vi "pulse detector on usrp host.vi"() -> ()   [LabVIEW 2021]
doc: "This template is for the Simple NI-USRP Streaming design, a design that shows the basics of streaming data to and from an NI USRP-294x/295x device. Refer to the block diagram for more information about how to use this template."
uses:
  FPGA/reciver params.ctl
  Host/SubVIs/Start Trigger.ctl
  <vilib>/userDefined/Silver/nirio_resource_slv.ctl
  Host/SubVIs/Streaming Xvcr FPGA Ref.ctl
  FPGA/PDW interpoter params.ctl
  Host/SubVIs/Initiate and Fetch (Multi).vi
  Host/SubVIs/Initiate and Fetch Time (Multi).vi
  Host/SubVIs/Initiate and Trigger.vi
  Host/SubVIs/Fetch Rx Data.vi
  Host/SubVIs/Fetch Rx Data (CDB WDT).vi
  Host/SubVIs/Check Aurora Link.vi
  Host/SubVIs/Check Stream Status.vi
  <vilib>/Utility/error.llb/Error Cluster From Error Code.vi
  <vilib>/rvi/errors/niLvFpgaAdjustHostInterfaceError.vi
  <vilib>/rvi/interface/nirviMethod/nirviMethod.xnode
  <vilib>/rvi/interface/nirviReadWriteControl/nirviReadWriteControl.xnode
  <vilib>/FPGAPlugInAG/Dynamic/niLvFpga_ReadFifo_Dynamic.vi
  <vilib>/rvi/errors/niLvFpgaMergeErrorWithErrorCode.vi
  NiFpgaLv.dll
  <vilib>/rvi/interface/Simulation/niFpgaSimulationCallBeginRW.vi
panel:
  in  "Tab Control":enum32{"sumorry", "Rx graphs"}(tab)
  in  "detection bar (dB)":dbl format="%#_3p"
  out "amp(dB)/ frequncy (Hz)":cluster{dbl[], dbl[]}(graph)
  out "amp(dB)":cluster{dbl[], dbl[]}(graph)
  out "F (Hz)":cluster{dbl[], dbl[]}(graph)
  out "PW":cluster{dbl[], dbl[]}(graph)
  out "mun of polses detected":i32
  out "spots from start":i32
  out "pulse rate (PPS)":dbl format="%#_6p"
  in  "base frequnce showen":bool
  in  "sample rate":dbl=200000000.0 format="%#_6p"
  in  "frequency":dbl=800000000.0 format="%#_6p"
  in  "pre amp":dbl=30.0
  in  "PW low bar":dbl
  in  "min AMP":dbl format="%#_3p"
  in  "Pw high bar":dbl=30000.0 format="%#_3g"
  in  "lo likege removal (#of bins)":i32
  out "PW_resolotion":dbl format="%#_6p"
  out "frequncy resolotion":dbl format="%#_3p"
  in  "reciver_params":T1={"min PW (fft cycels)"=0, "max PW (fft cycels)"=1500, "max gap (fft cycels)"=0, "detection bar (liniar amp)"=93.0, "peak detect"=FALSE}
  out "acquiring":bool caption="Streaming"
  in  "Stop":bool
  # "pulse detector on usrp"
  # "this application runs the pulse detector on the IQ stream inside the USRP.\nset the parameters and run it.\nthe reciver params are the parameters needed for the pulse detector:\n max gap - the maxiemom of undetected parts in the spot that \nthe detector keep loking for continuety.\nRx max PW - if the pulse is CW then we like to get  a PDW even if the pulse isnt done.\nRx min PW - less then this size is probbly just termal noise\nRx detection bar - the detection bar.\ndisplay filters could help the user make the presenting graphs easyer to understend."
  # "user filter"
  # "USRP setup"
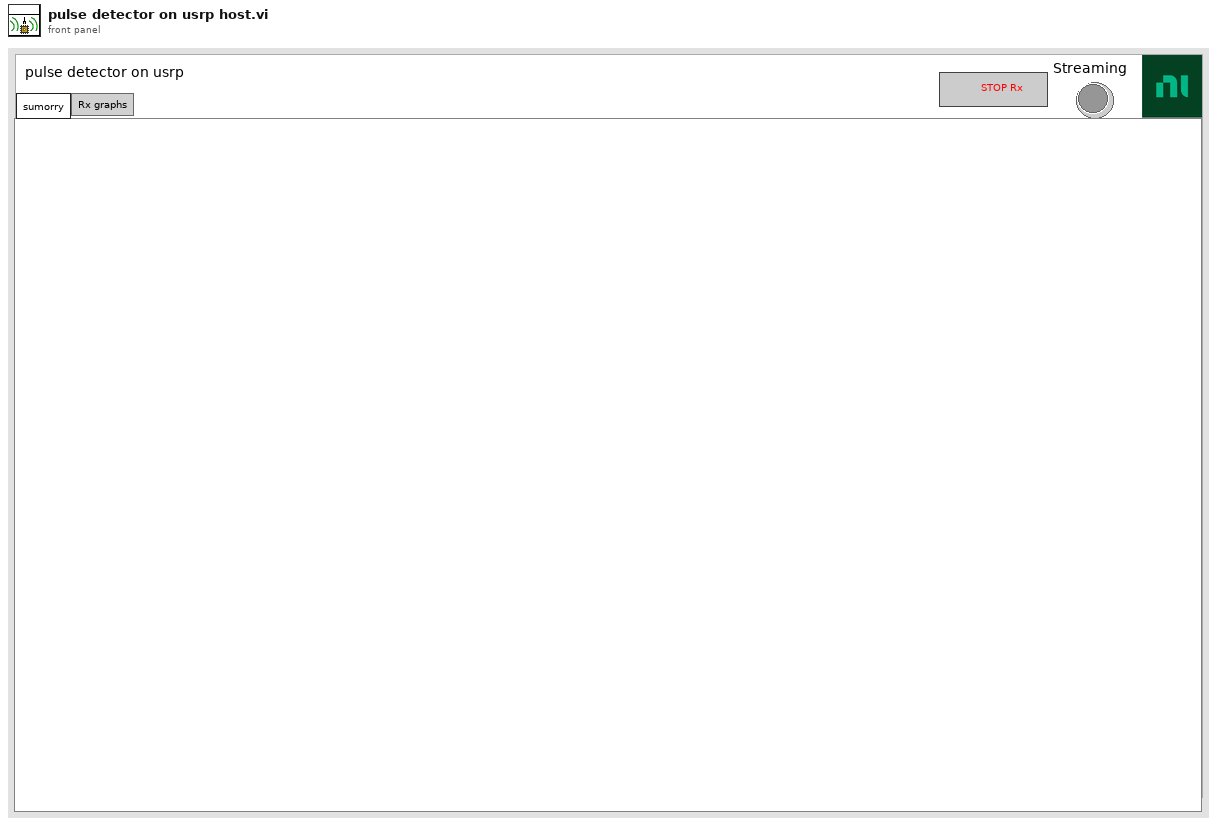
[diagram p1: front panel]
types:
  T1 = typedef "reciver params.ctl" = cluster{"min PW (fft cycels)":u16, "max PW (fft cycels)":u16, "max gap (fft cycels)":u8, "detection bar (liniar amp)":fxp<+,64,63>, "peak detect":bool}
  T2 = typedef "nirio_resource_slv.ctl" = tag
  T3 = typedef "Start Trigger.ctl" = enum8{"Software", "Digital Edge", "Rx Start Trigger", "Tx Start Trigger", "Immediate", "Future Time Event"}
  T4 = cluster{"rf enable 0":bool, "rf config 0":cluster{"antenna":string, "frequency":dbl, "lo frequency":dbl, "level":dbl}, "rf enable 1":bool, "rf config 1":cluster{"antenna":string, "frequency":dbl, "lo frequency":dbl, "level":dbl}, "transfer mode":enum16{"Finite", "Continuous"}, "sample rate":dbl, "number of samples":u32, "start trigger":T3}
  T5 = enum16{"open", "open or create", "create or replace", "create", "open (read-only)"}
  T6 = typedef "Rx Channels.ctl" = cluster{"rx config":cluster{"channel configuration":cluster{"channel enable":bool, "channel configuration":cluster{"antenna":string, "frequency":dbl, "lo frequency":dbl, "level":dbl}}[], "transfer mode":enum16{"Finite", "Continuous"}, "sample rate":dbl, "number of samples":u32, "start trigger":T3}, "reference frequency source":string, "rx.data sink":enum16{"SFP Port 0", "SFP Port 1", "Host"}, "rx.enabled channels":string[], "vertical range":dbl[], "rx.coerced configurations":cluster{"coerced frequencies":dbl[], "coerced lo frequencies":dbl[], "coerced levels":dbl[], "coerced sample rates":dbl[]}}
  T7 = typedef "niUsrpRio Config v1 Host.lvlib/niUsrpRio Session.ctl" = cluster{"FPGA Interface":refnum<k20>, "RIO Interface Number":u32, "Data Clock Rate":u32, "FPGA Data Clock Rate":u32, "Global Settings Register Bus":T8, "Radio 0 Settings Register Bus":T8, "Radio 1 Settings Register Bus":T8, "Radio Settings Bus Semaphore":T9, "DB Queues":T10[], "Characterization Data Valid?":bool, "EEPROM Header":T11, "Device Data Header":T12, "EEPROM Characterization Header":T13, "Characterization Data":T14[], "FPGA Current Version":u32, "FPGA Oldest Compatible Version":u32, "Fixed Logic Current Version":u32, "Fixed Logic Oldest Compatible Version":u32, "FPGA Radio Settings Bus Current Version":u32, "FPGA Radio Settings Bus Oldest Compatible Version":u32, "FPGA Board Config Current Version":u32, "FPGA Board Config Oldest Compatible Version":u32, "Daughterboard Clock Rate":u32, "daughterboard configuration session handles":u64[]}
  T8 = typedef "niInstr Register Bus v0 Host.lvlib/Register Bus Session.ctl" = refnum<queue>
  T9 = typedef "Semaphore RefNum" = refnum<k1>
  T10 = typedef "niUsrpRio Config v1 Host.lvlib/DB Queue Reference.ctl" = refnum<queue>
  T11 = typedef "niUsrpRio Config v1 Host.lvlib/EEPROM Header.ctl" = cluster{"Checksum":u32, "Product Code":u16, "Hardware Current Version":u16, "Hardware Oldest Compatible Version":u16, "EEPROM Map Current Version":u16, "EEPROM Map Oldest Compatible Version":u16, "User Password":string, "Pointer to Factory Header":u32, "Pointer to User Header":u32, "Recommended Interval":u16, "Number of Reserved Bytes":i32, "Number of Daughterboards":u8, "Daughterboard IDs":u16[], "Daughterboard Serial Numbers":string[]}
  T12 = typedef "niUsrpRio Config v1 Host.lvlib/EEPROM Device Data Header.ctl" = cluster{"Checksum":u32, "Number of Channels":u8, "Number of Gain Settings":u16[], "Pointer to Characterization Data":u32[], "Number of Reserved Bytes":i32, "Number of Frequencies":u16[]}
  T13 = typedef "niUsrpRio Config v1 Host.lvlib/EEPROM Characterization Header.ctl" = cluster{"Checksum":u32, "Date":timestamp, "Temperature":sgl, "Misc. Info":string, "Pointer to Device Data Header":u32, "Number of Reserved Bytes":i32}
  T14 = typedef "niUsrpRio Config v1 Host.lvlib/Characterization Data.ctl" = cluster{"Gains[dB]":dbl[], "Frequencies [Hz]":dbl[], "IQ Imbalance Table":T15[], "Measured Gains[dB]":dbl[][]}
  T15 = typedef "niUsrpRio Config v1 Host.lvlib/IQ Imbalance.ctl" = cluster{"Gain Imbalance [linear]":dbl, "Phase Imbalance [radians]":dbl, "Offset":cdb}
  T16 = typedef "PDW interpoter params.ctl" = cluster{"Fs (Hz)":u32, "fft size ":u32, "F base (Hz)":u32, "min AMP (dB)":dbl, "PW low bar (fft cycle)":dbl, "Pw high bar (fft cycle)":dbl, "lo likege removal (fft bin)":i32, "max gap (fft cycle)":dbl}
  T17 = typedef "Streaming Xvcr FPGA Ref.ctl" = refnum<k20>
  T18 = cluster{"rx.state":enum16{"Idle", "Active"}, "rx.samples processed":u32, "rx.number of fifo overflows":u32, "rx.number of iq data overflows":u64[], "rx.dsp reset done":bool}
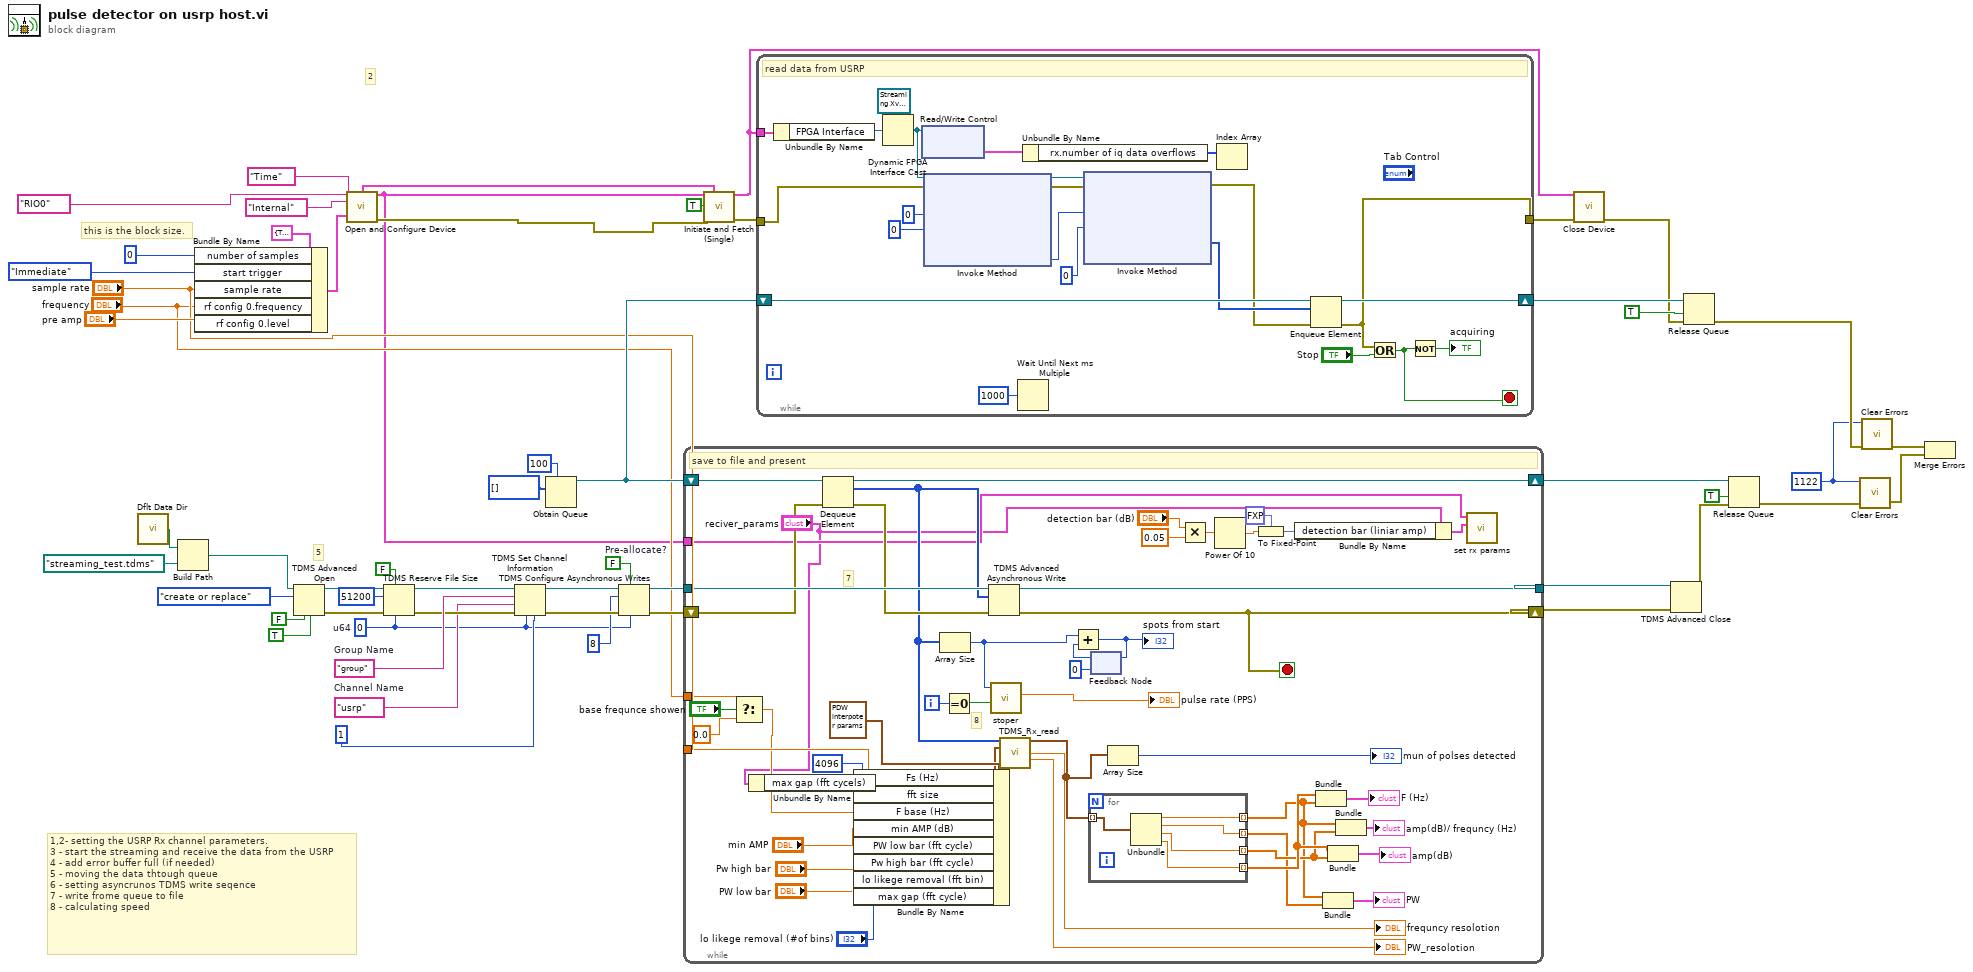
[diagram p0: block diagram]
diagram:
  w22 = 1122 ("specific error code to clear (0: all)")
  w46 = FALSE  # Pre-allocate?
  w37 = u64 0  # u64
  w55 = "group"  # Group Name
  w39 = "usrp"  # Channel Name
  # "2"
  # "this is the block size."
  # "1,2- setting the USRP Rx channel parameters.\n3 - start the streaming and receive the data from the USRP\n4 - add error buffer full (if needed)\n5 - moving the data thtough queue   \n6 - setting asyncrunos TDMS write seqence\n7 - write frome queue to file\n8 - calculating speed"
  # "5"
  n1 = call <vilib>:"Dflt Data Dir.vi"() -> ("App:Default Data Directory"=w32:path)
  n2 = Build Path(base path=w32, name or relative path=path "streaming_test.tdms") -> (appended path=w31:path)
  n3 = Bundle By Name(cluster=T4 {"rf enable 0"=TRUE, "rf config 0"={"antenna"="RX1", "frequency"=2000000000.0, "lo frequency"=-1.0, "level"=0.0}, "rf enable 1"=FALSE, "rf config 1"={"antenna"="RX2", "frequency"=2000000000.0, "lo frequency"=-1.0, "level"=0.0}, "transfer mode"=enum."Continuous", "sample rate"=10000000.0, "number of samples"=4194304, "start trigger"=enum."Immediate"} ("rx config"), "number of samples"=0, "start trigger"=Start_Trigger."Immediate", "sample rate"="sample rate", "rf config 0.frequency"="frequency", "rf config 0.level"="pre amp") -> (w15:T4)
  n4 = TDMS Advanced Open(4:TRUE ("enable asynchronous? (T)"), 6:FALSE ("disable buffering? (T)"), 10:T5."create or replace" ("operation (0:open)"), 11:w31) -> (0:w51:errorcluster, 3:w52:refnum<k34>)  [unwired: 1 in, 1 out]
  n5 = call "Open and Configure Device.vi"("USRP RIO Device"=T2 "RIO0" ("USRP RIO device"), "reference frequency source"="Internal", "which bitfile"="Time", "rx config"=w15) -> ("rx channels"=w8:T6, "niUsrpRio Session (out)"=w1:T7, "error out"=w2:errorcluster)  [unwired: 5 in, 4 out]
  n6 = TDMS Reserve File Size(6:w37, 7:FALSE ("append? (T)"), 8:w51, 10:u64 51200 ("reserve size"), 11:w52) -> (0:w49:errorcluster, 3:w50:refnum<k34>)
  n7 = TDMS Set Channel Information(4:u32 1 ("y"), 6:w37, 8:w49, 9:w39, 10:w55, 11:w50) -> (0:w48:errorcluster, 3:w47:refnum<k34>)  [unwired: 1 in]
  n8 = Obtain Queue(max queue size (-1, unlimited)=100, element data type=u64[] [] ("waveform data")) -> (queue out=w23:refnum<queue>)  [unwired: 3 in, 2 out]
  n9 = TDMS Configure Asynchronous Writes(6:w37, 7:w46, 8:w48, 10:u32 8 ("max asynchronous writes (4)"), 11:w47) -> (0:w40:errorcluster, 3:w43:refnum<k34>)  [unwired: 2 in]
  n10 = while {
    tunnel: w43 -> [w103]
    shift-right: [w99] -> w41
    shift-left: w23 -> [w104]
    tunnel: [w101] -> w42
    shift-right: [w102] -> w35
    shift-left: w40 -> [w98]
    tunnel: "sample rate" -> [w69]
    tunnel: "frequency" -> [w67]
    tunnel: w1 -> [w60]
    i -> [w100]
    stop <- w102 stop-if-true
    # "8"
    # "7"
    # "save to file and present"
    n11 = Select(t=w67, s="base frequnce showen", f=0.0) -> (s? t:f=w68:dbl)
    n12 = Unbundle By Name("reciver_params") -> ("max gap (fft cycels)"=w74:u8)
    n13 = Dequeue Element(queue=w104, error in (no error)=w98) -> (queue out=w99:refnum<queue>, element=w79:u64[], error out=w97:errorcluster)  [unwired: 1 in, 1 out]
    n14 = Bundle By Name(cluster=T16 {"Fs (Hz)"=200000000, "fft size "=4096, "F base (Hz)"=2000000000, "min AMP (dB)"=0.0, "PW low bar (fft cycle)"=0.0, "Pw high bar (fft cycle)"=7000.0, "lo likege removal (fft bin)"=-1, "max gap (fft cycle)"=0.0} ("PDW interpoter params"), "Fs (Hz)"=w69, "fft size"=u32 4096, "F base (Hz)"=w68, "min AMP (dB)"="min AMP", "PW low bar (fft cycle)"="PW low bar", "Pw high bar (fft cycle)"="Pw high bar", "lo likege removal (fft bin)"="lo likege removal (#of bins)", "max gap (fft cycle)"=w74) -> (w76:T16)
    n15 = Array Size(array=w79) -> (size(s)=w94:i32)
    n16 = Equal To 0?(x=w100) -> (x = 0?=w96:bool)
    n17 = TDMS Advanced Asynchronous Write(8:w97, 10:w79, 11:w103) -> (0:w102:errorcluster, 3:w101:refnum<k34>)
    n18 = call "stoper.vi"("start"=w96, "x mission"=w94) -> ("x rate"=→"pulse rate (PPS)":dbl)  [unwired: 7 in, 2 out]
    n19 = call "TDMS_Rx_read.vi"("Array in"=w79, "PDW interpoter params"=w76) -> ("Array"=w80:cluster{dbl, dbl, "fixed-point":dbl, dbl}[], "frequncy resolotion"=→"frequncy resolotion":dbl, "PW_resolotion"=→"PW_resolotion":dbl)  [unwired: 11 in]
    n20 = for {
      tunnel: w80 -> [w109] mode=indexing
      tunnel: [w108] -> w78 mode=indexing
      tunnel: [w107] -> w81 mode=indexing
      tunnel: [w106] -> w82 mode=indexing
      tunnel: [w105] -> w83 mode=indexing
      n21 = Unbundle(w109) -> (w108:dbl, w107:dbl, "fixed-point"=w106:dbl, w105:dbl)
    }
    n22 = feedback #1(0) -> (w92:i32)
    n23 = Add(x=w94, y=w92) -> (x+y=w93:i32)
    "spots from start" <- w93
    n24 = feedback-in #1(w93) -> ()
    n25 = Array Size(array=w80) -> (size(s)=→"mun of polses detected":i32)
    n26 = Multiply(x="detection bar (dB)", y=0.05) -> (x*y=w61:dbl)
    n27 = Power Of 10(x=w61) -> (10^x=w62:dbl)
    n28 = To Fixed-Point(fixed-point type=fxp<+,64,63> 0.0 ("detection bar (liniar amp)"), number=w62) -> (fixed-point=w63:fxp<+,64,63>)
    n29 = Bundle By Name(cluster="reciver_params", "detection bar (liniar amp)"=w63) -> (w64:T1)
    n30 = Bundle(w83, w78) -> (→"F (Hz)":cluster{dbl[], dbl[]})  [unwired: 1 in]
    n31 = Bundle(w78, w81) -> (→"PW":cluster{dbl[], dbl[]})  [unwired: 1 in]
    n32 = Bundle(w83, w82) -> (→"amp(dB)":cluster{dbl[], dbl[]})  [unwired: 1 in]
    n33 = Bundle(w78, w82) -> (→"amp(dB)/ frequncy (Hz)":cluster{dbl[], dbl[]})  [unwired: 1 in]
    n34 = call "set rx params.vi"("reciver_params"=w64, "niUsrpRio Session (out)"=w60) -> ()  [unwired: 8 in, 2 out]
  }
  n35 = call "Initiate and Fetch (Single).vi"("niUsrpRio Session"=w1, "rx channels"=w8, "first iteration"=TRUE, "error in"=w2) -> ("niUsrpRio Session (out)"=w7:T7, "error out"=w6:errorcluster)  [unwired: 9 in, 1 out]
  n36 = while {
    shift-right: [w131] -> w29
    shift-left: w23 -> [w130]
    tunnel: [w126] -> w13
    tunnel: w7 -> [w121]
    tunnel: w6 -> [w113]
    stop <- w127 stop-if-true
    # "read data from USRP"
    n37 = Unbundle By Name(w121) -> ("FPGA Interface"=w125:refnum<k20>)
    n38 = Dynamic FPGA Interface Cast(Session In=T17 refnum ("Type"), Type=w125) -> (Session Out=w115:T17)
    n39 = xnode "Read/Write Control"("FPGA VI Reference In"=w115) -> ("rx.status"=w123:T18)  [unwired: 1 in, 2 out]
    n40 = xnode "Invoke Method"("FPGA VI Reference In"=w115, "error in"=w113, "Number of Elements"=u32 0, "Timeout (ms)"=0) -> ("FPGA VI Reference Out"=w111:T17, "error out"=w114:errorcluster, "Elements Remaining"=w120:u32)  [unwired: 1 out]
    n41 = Wait Until Next ms Multiple(millisecond multiple=u32 1000) -> ()  [unwired: 1 out]
    n42 = Unbundle By Name(w123) -> ("rx.number of iq data overflows"=w122:u64[])
    n43 = xnode "Invoke Method"("FPGA VI Reference In"=w111, "error in"=w114, "Number of Elements"=w120, "Timeout (ms)"=0) -> ("error out"=w112:errorcluster, "Data"=w117:u64[])  [unwired: 2 out]
    n44 = Index Array(array=w122) -> ()  [unwired: 1 in, 1 out]
    n45 = Enqueue Element(queue=w130, element=w117, error in (no error)=w112) -> (queue out=w131:refnum<queue>, error out=w126:errorcluster)  [unwired: 1 in, 1 out]
    n46 = Or(x=w126, y="Stop") -> (x .or. y?=w127:bool)
    n47 = Not(x=w127) -> (.not. x?=→"acquiring":bool)
  }
  n48 = call "Close Device.vi"("niUsrpRio Session"=w7, "error in"=w13) -> ("error out"=w14:errorcluster)  [unwired: 13 in]
  n49 = TDMS Advanced Close(8:w35, 11:w42) -> (0:w30:errorcluster)  [unwired: 2 in, 1 out]
  n50 = Release Queue(queue=w29, force destroy? (F)=TRUE, error in (no error)=w14) -> (error out=w25:errorcluster)  [unwired: 2 out]
  n51 = Release Queue(queue=w41, force destroy? (F)=TRUE, error in (no error)=w30) -> (error out=w24:errorcluster)  [unwired: 2 out]
  n52 = call <vilib>:"Clear Errors.vi"("error in (no error)"=w24, "specific error code to clear (0: all)"=w22) -> ("error out"=w21:errorcluster)  [unwired: 4 in, 1 out]
  n53 = call <vilib>:"Clear Errors.vi"("error in (no error)"=w25, "specific error code to clear (0: all)"=w22) -> ("error out"=w26:errorcluster)  [unwired: 4 in, 1 out]
  n54 = Merge Errors(w26, w21) -> ()  [unwired: 1 out]
